vi "Update UI Interlock.vi"(8 "error in (no error)":errorcluster, 11 "Thermal Chamber Controller In":refnum<class "Thermal Chamber Controller.lvclass">) -> (0 "error out":errorcluster, 3 "Thermal Chamber Controller Out":refnum<class "Thermal Chamber Controller.lvclass">)   [LabVIEW 2020, in "Thermal Chamber Controller.lvclass"]
uses:
  Thermal Chamber Controller.lvclass
  <vilib>/Asteme/Triarc Framework/Process/Process.lvclass/Process.ctl
  Thermal Chamber Controller.lvclass/Thermal Chamber Controller.ctl
  <vilib>/Utility/error.llb/Clear Errors.vi
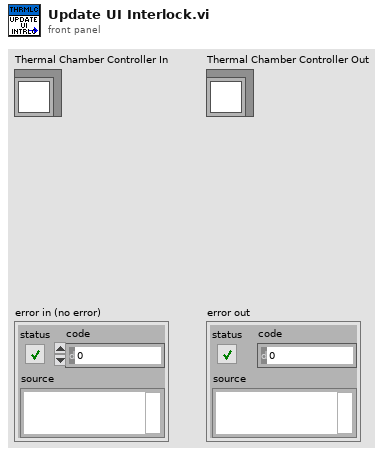
[diagram p1: front panel]
types:
  T1 = typedef "Thermal Chamber Controller.lvclass/Heater State.ctl" = enum16{"Heater Disabled", "Heater Enabled"}
  T2 = enum8{"Enabled", "Disabled", "Disabled and Grayed Out"}
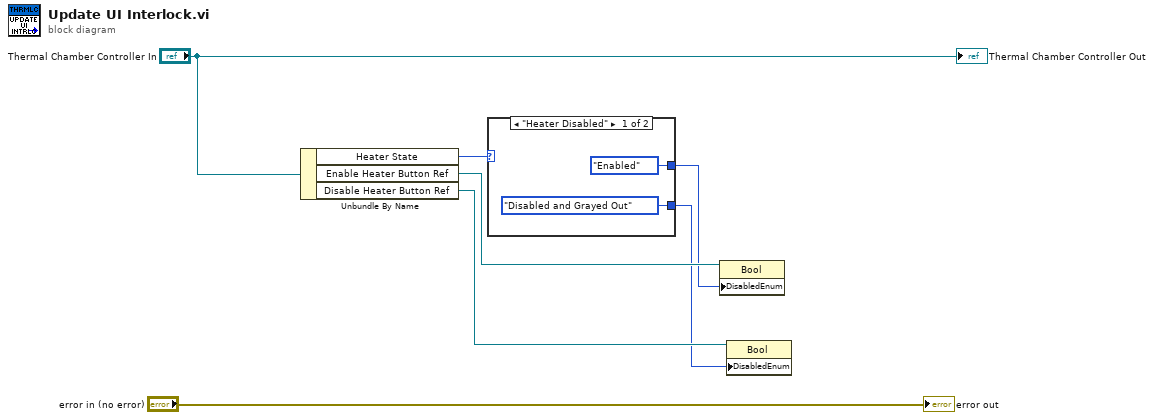
[diagram p0: block diagram]
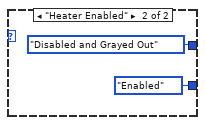
[diagram p2: hidden frame]
diagram:
  n1 = Unbundle By Name("Thermal Chamber Controller In") -> ("Heater State"=w4:T1, "Enable Heater Button Ref"=w5:refnum<vi>, "Disable Heater Button Ref"=w3:refnum<vi>)
  n2 = case shown="\"Heater Disabled\"" w4 {
    tunnel: [T2."Enabled" ("Disabled") T2."Disabled and Grayed Out" ("Disabled")] -> w2
    tunnel: [T2."Disabled and Grayed Out" ("Disabled") T2."Enabled" ("Disabled")] -> w1
    frame "Heater Disabled" {
    }
    frame "Heater Enabled" {
    }
  }
  n3 = property class="Bool"(reference=w5, "DisabledEnum"=w2) -> ()  [unwired: 1 in, 2 out]
  n4 = property class="Bool"(reference=w3, "DisabledEnum"=w1) -> ()  [unwired: 1 in, 2 out]
  "error out" <- "error in (no error)"
  "Thermal Chamber Controller Out" <- "Thermal Chamber Controller In"
